vi "00 Main (single phase) (2017).vi"() -> ()   [LabVIEW 2017]
uses:
  <vilib>/DAQmx/read.llb/DAQmx Read (Analog 1D Wfm NChan NSamp).vi
  <vilib>/DAQmx/miscellaneous.llb/DAQmx Fill In Error Info.vi
panel:
  out "Error out (DAQ Loop)":errorcluster
  out "DAQ Loop Iterations":i32
  out "Raw DAQ Output":dynamicdata(graph)=[{"t0"=timestamp(3367839419.335167 s since 1904-01-01), "dt"=0.00016666666666666663, "Y"=array[240 elements], "attributes"=variant("NI_ChannelName"=variant(string "Voltage_0"), "NI_UnitDescription"=variant(string "Volts"))}, {"t0"=timestamp(3367839419.3351874 s since 1904-01-01), "dt"=0.00016666666666666663, "Y"=array[240 elements], "attributes"=variant("NI_ChannelName"=variant(string "Voltage_1"), "NI_UnitDescription"=variant(string "Volts"))}, {"t0"=timestamp(3367839419.3352084 s since 1904-01-01), "dt"=0.00016666666666666663, "Y"=array[240 elements], "attributes"=variant("NI_ChannelName"=variant(string "Voltage_2"), "NI_UnitDescription"=variant(string "Volts"))}]
  in  "All Stop!":bool
  out "Frequency 2":dynamicdata(graph) caption="Frequency"
  out "Phase 2":dynamicdata(graph) caption="Frequency"
  out "Frequency":dbl format="%.2f"
  out "Amplitude":dbl format="%.2f"
  out "Phase":dbl format="%.2f"
  out "Acquisition Time":timestamp
  out "Voltage Waveform":dynamicdata(graph)=[{"t0"=timestamp(3377170241.8512917 s since 1904-01-01), "dt"=0.00016666666666666663, "Y"=array[300 elements]}, {"t0"=timestamp(3377170241.8513126 s since 1904-01-01), "dt"=0.00016666666666666663, "Y"=array[300 elements]}, {"t0"=timestamp(3377170241.8513336 s since 1904-01-01), "dt"=0.00016666666666666663, "Y"=array[300 elements]}]
  out "IP":string
  out "Port":i32
  out "Transmitted Data":string
  out "Stop":bool
  out "Elements in Acquisition Buffer":i32
  # "V1.2 - PFI0 (Single Phase)"
  # "50.5"
  # "The code and design of this VI are licensed \nunder the terms of the New BSD License.\nPlease see the VI documentation or License.txt\nfor more details.\n\nCopyright (c) 2012, David Laverty\nwww.OpenPMU.org"
  # "Configuration Information:\n\nThe ID and IP address to which the OpenPMU sends data is configured by 'C:\\PMUconfig.ini'.  If this doesn't exist, create it.\n\nCopy and paste the blue text below without the dashed lines into PMUconfig.ini.\n\n[Telecoms]\nID=PMU123\nIP=192.168.1.100\nPort=40001\n\nIP and Port may be any values within normal IPv4 range.  ID should be six alpha-numeric characters."
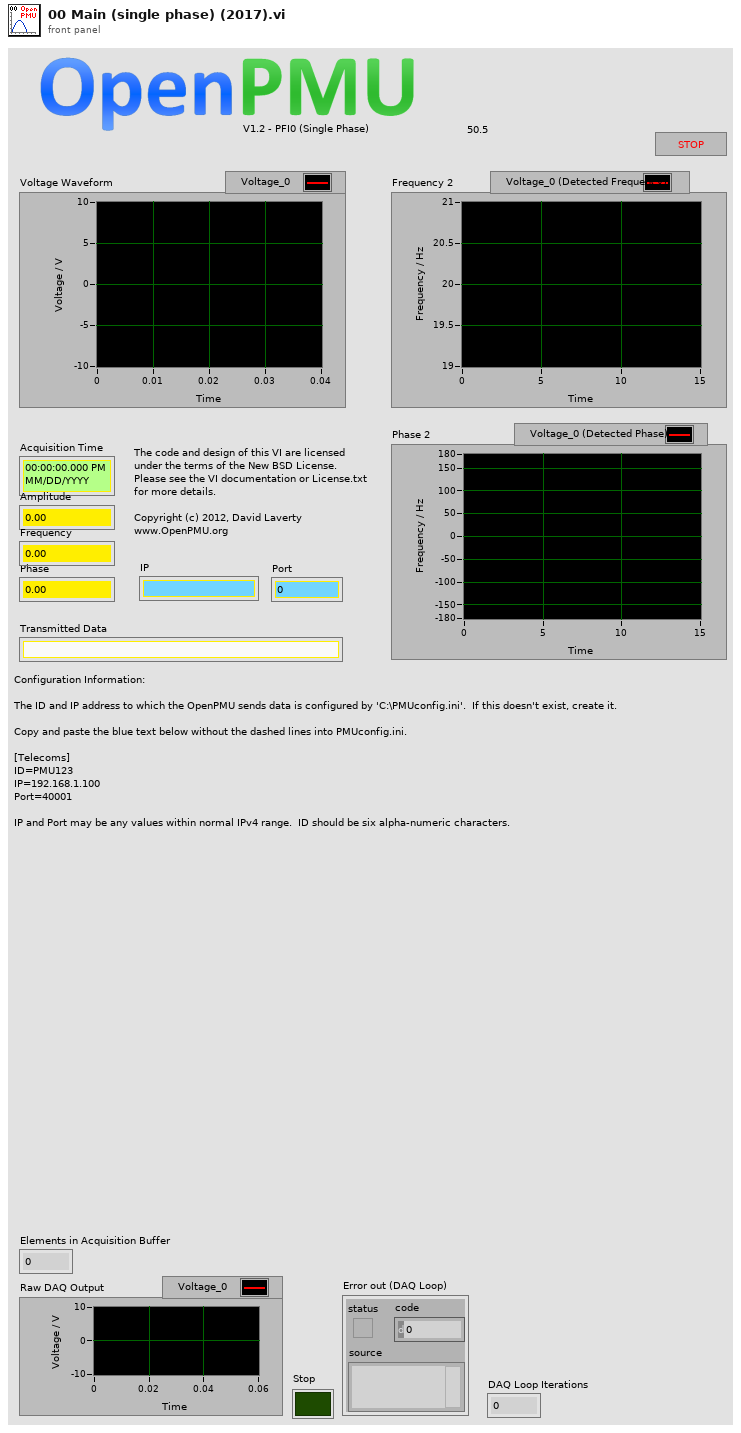
[diagram p1: front panel]
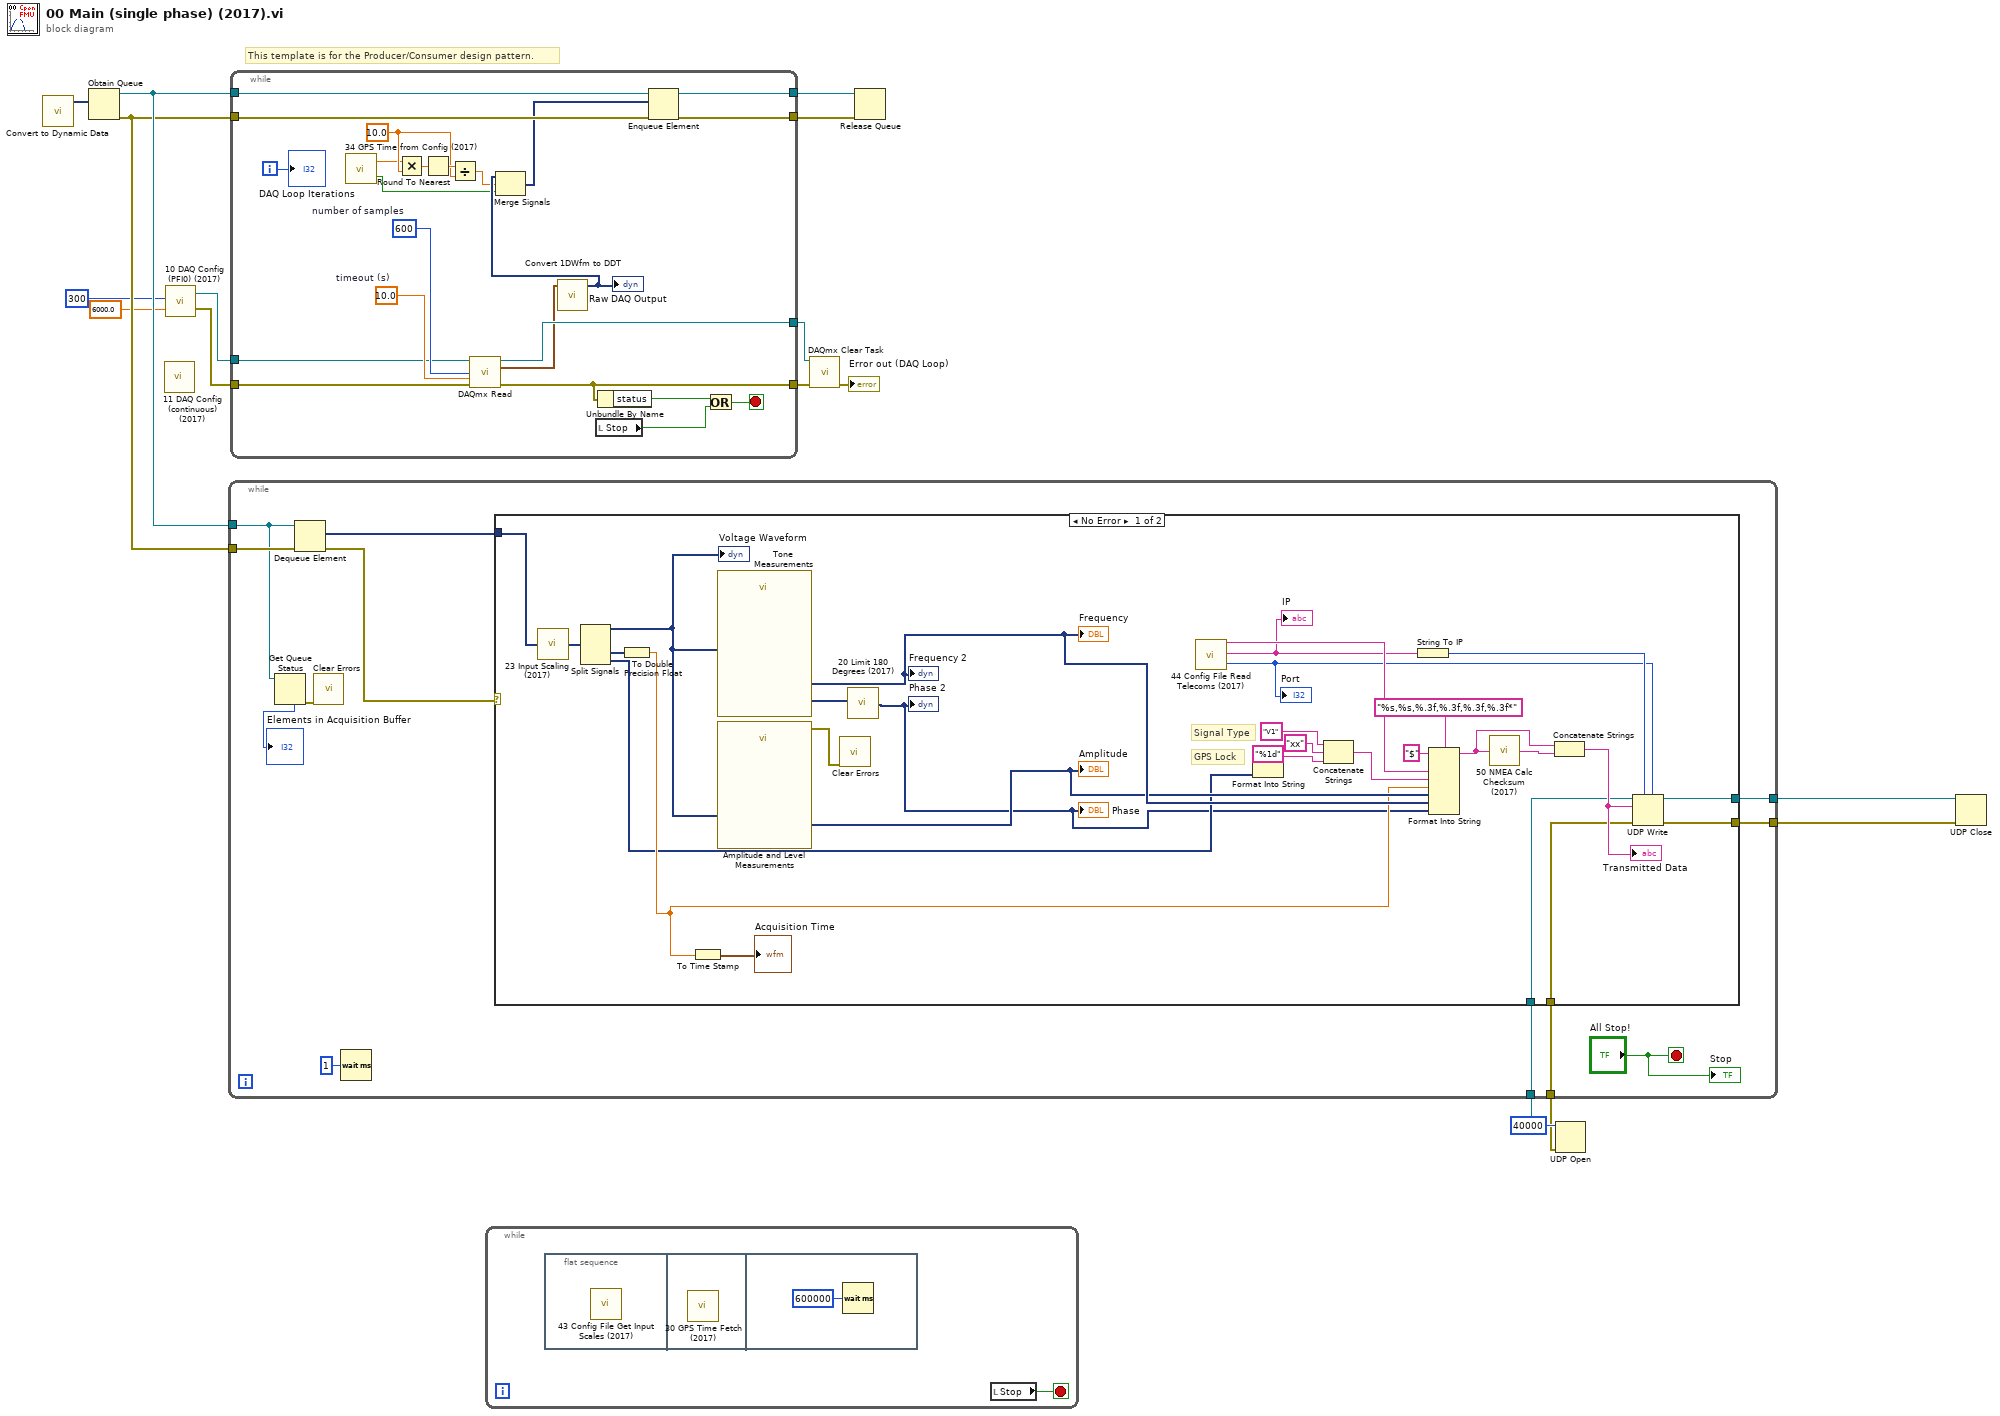
[diagram p0: block diagram]
diagram:
  # "This template is for the Producer/Consumer design pattern."
  n1 = call "Convert to Dynamic Data"() -> ("Dynamic Data Type"=w14:dynamicdata)  [unwired: 4 in]
  n2 = Obtain Queue(element data type=w14) -> (queue out=w11:refnum<queue>, error out=w10:errorcluster)  [unwired: 4 in, 1 out]
  n3 = call "11 DAQ Config (continuous) (2017).vi"() -> ()  [unwired: 1 in, 2 out]
  n4 = call "10 DAQ Config (PFI0) (2017).vi"("rate"=6000.0, "number of samples"=300) -> ("Error Out"=w1:errorcluster, "task out"=w2:refnum<k21>)  [unwired: 1 in]
  n5 = while {
    tunnel: w1 -> [w26]
    tunnel: w2 -> [w27]
    tunnel: [w37] -> w17
    tunnel: [w36] -> w16
    tunnel: w11 -> [w31]
    tunnel: w10 -> [w30]
    tunnel: [w29] -> w13
    tunnel: [w28] -> w12
    i -> [w35]
    stop <- w34 stop-if-true
    w20 = 10.0 ("y")
    w38 = 10.0  # timeout (s)
    w40 = 600  # number of samples
    n6 = call "34 GPS Time from Config (2017).vi"() -> ("GPS Lock"=w18:bool, "Time"=w19:dbl)  [unwired: 2 in]
    n7 = Multiply(x=w19, y=w20) -> (x*y=w23:dbl)
    n8 = Round To Nearest(number=w23) -> (nearest integer value=w22:dbl)
    n9 = Divide(x=w22, y=w20) -> (x/y=w21:dbl)
    n10 = call-poly <vilib>:"DAQmx Read.vi"("task/channels in"=w27, "number of samples per channel"=w40, "timeout"=w38, "error in"=w26) -> ("task out"=w37:refnum<k21>, "data"=w33:waveform(dbl)[], "error out"=w36:errorcluster)  [unwired: 9 in]
    n11 = call <vilib>:"Convert 1DWfm to DDT.vi"("Array of Waveforms"=w33) -> ("Dynamic Data Type"=w25:dynamicdata)  [unwired: 3 in]
    "Raw DAQ Output" <- w25
    n12 = Merge Signals(w25, w21, w18) -> (w24:dynamicdata)
    n13 = local read "Stop"() -> (w32:bool)
    n14 = Unbundle By Name(w36) -> ("status"=w39:bool)
    n15 = Enqueue Element(queue=w31, element=w24, error in (no error)=w30) -> (queue out=w29:refnum<queue>, error out=w28:errorcluster)  [unwired: 1 in, 1 out]
    n16 = Or(x=w39, y=w32) -> (x .or. y?=w34:bool)
    "DAQ Loop Iterations" <- w35
  }
  n17 = while {
    stop <- w41 stop-if-true
    n18 = flat-sequence {
      frame #0 {
        n19 = call "43 Config File Get Input Scales (2017).vi"() -> ()  [unwired: 1 in]
      }
      frame #1 {
        n20 = call "30 GPS Time Fetch (2017).vi"() -> ()  [unwired: 1 in]
      }
      frame #2 {
        n21 = Wait (ms)(milliseconds to wait=u32 600000) -> ()  [unwired: 1 out]
      }
    }
    n22 = local read "Stop"() -> (w41:bool)
  }
  n23 = call <vilib>:"DAQmx Clear Task.vi"("task in"=w17, "error in"=w16) -> ("error out"=→"Error out (DAQ Loop)":errorcluster)  [unwired: 13 in]
  n24 = Release Queue(queue=w13, error in (no error)=w12) -> ()  [unwired: 1 in, 3 out]
  n25 = UDP Open(11:u16 40000 ("port")) -> (port=w8:refnum<k16>, 0:w7:errorcluster)  [unwired: 4 in, 1 out]
  n26 = while {
    tunnel: w11 -> [w48]
    tunnel: w10 -> [w50]
    tunnel: w8 -> [w47]
    tunnel: w7 -> [w46]
    tunnel: [w45] -> w6
    tunnel: [w44] -> w5
    stop <- "All Stop!" stop-if-true
    n27 = Get Queue Status(queue=w48) -> (error out=w43:errorcluster, # elements in queue=→"Elements in Acquisition Buffer":i32)  [unwired: 2 in, 6 out]
    n28 = Dequeue Element(queue=w48, error in (no error)=w50) -> (element=w51:dynamicdata, error out=w52:errorcluster)  [unwired: 1 in, 2 out]
    n29 = call <vilib>:"Clear Errors.vi"("error in (no error)"=w43) -> ()  [unwired: 5 in, 2 out]
    n30 = Wait (ms)(milliseconds to wait=u32 1) -> ()  [unwired: 1 out]
    n31 = case shown="No Error" w52 {
      tunnel: w51 -> [w63 _]
      tunnel: w47 -> [w78 w86]
      tunnel: w46 -> [w77 w85]
      tunnel: [w76 w86] -> w45
      tunnel: [w75 w85] -> w44
      frame No Error {
        # "GPS Lock"
        # "Signal Type"
        n32 = call "23 Input Scaling (2017).vi"("Input (Raw)"=w63) -> ("Output (Scaled)"=w62:dynamicdata)
        n33 = Split Signals(w62) -> (w74:dynamicdata, w73:dynamicdata, w69:dynamicdata)  [unwired: 5 in, 2 out]
        "Voltage Waveform" <- w74
        n34 = To Double Precision Float(number=w73) -> (double precision float=w70:dbl)
        n35 = To Time Stamp(1:w70) -> (0:→"Acquisition Time":timestamp)
        n36 = call "Tone Measurements"("Signals"=w74) -> ("Phase"=w61:dynamicdata, "Frequency"=w72:dynamicdata)  [unwired: 7 in, 2 out]
        "Frequency 2" <- w72
        "Frequency" <- w72
        n37 = call "Amplitude and Level Measurements"("Signals"=w74) -> ("Cycle RMS"=w71:dynamicdata, "error out"=w84:errorcluster)  [unwired: 13 in]
        "Amplitude" <- w71
        n38 = call <vilib>:"Clear Errors.vi"("error in (no error)"=w84) -> ()  [unwired: 5 in, 2 out]
        n39 = call "20 Limit 180 Degrees (2017).vi"("Angle In"=w61) -> ("Angle Out"=w60:dynamicdata)
        "Phase 2" <- w60
        "Phase" <- w60
        n40 = call "44 Config File Read Telecoms (2017).vi"() -> ("Port"=w57:i32, "IP"=w58:string, "ID"=w59:string)  [unwired: 3 in]
        "IP" <- w58
        "Port" <- w57
        n41 = Format Into String(format string="%1d", w69) -> (resulting string=w64:string)  [unwired: 2 in, 1 out]
        n42 = Concatenate Strings("V1" ("input 2"), "xx" ("string"), w64) -> (w66:string)
        n43 = String To IP(1:w58) -> (0:w80:u32)
        n44 = Format Into String(format string="%s,%s,%.3f,%.3f,%.3f,%.3f*", initial string="$", w59, w66, w70, w71, w72, w60) -> (resulting string=w56:string)  [unwired: 1 in, 1 out]
        n45 = call "50 NMEA Calc Checksum (2017).vi"("GPS String"=w56) -> ("hex integer string"=w55:string)  [unwired: 1 in, 1 out]
        n46 = Concatenate Strings(w56, w55) -> (w79:string)
        "Transmitted Data" <- w79
        n47 = UDP Write(address=w80, port or service name=w57, connection ID=w78, data in=w79, 8:w77) -> (error out=w75:errorcluster, 3:w76:refnum<k16>)  [unwired: 1 in]
      }
      frame Error {
      }
    }
    "Stop" <- "All Stop!"
  }
  n48 = UDP Close(connection ID=w6, 8:w5) -> ()  [unwired: 2 out]
